vi "mouse_scroll_to_Z_3D.vi"(8 "Previous_Z":dbl, 10 "Scrolling":i32) -> (0 "Zmax":dbl=2.5, 2 "Z":dbl)   [LabVIEW 2011]
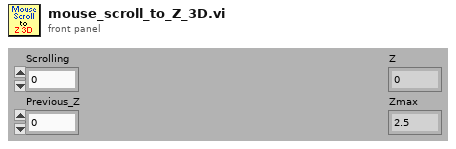
[diagram p1: front panel]
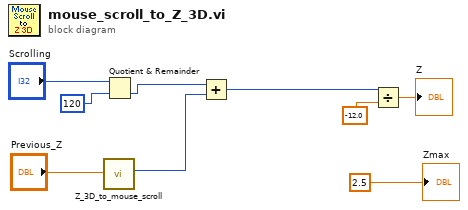
[diagram p0: block diagram]
diagram:
  n1 = call "Z_3D_to_mouse_scroll.vi"("Z"="Previous_Z") -> ("Scrolling"=w3:i32)  [unwired: 10 in]
  n2 = Quotient & Remainder(x="Scrolling", y=120) -> (floor(x/y)=w5:i32)  [unwired: 1 out]
  n3 = Add(x=w5, y=w3) -> (x+y=w2:i32)
  n4 = Divide(x=w2, y=-12.0) -> (x/y=→"Z":dbl)
  "Zmax" <- 2.5
